vi "河内塔.vi"() -> ()   [LabVIEW 2016]
panel:
  in  "等待时间（毫秒）":u32=200
  out "二维图片":picture
  out "C":u8[](array[numeric])
  out "B":u8[](array[numeric])
  out "A":u8[](array[numeric])=[1, 2, 3]
  out "数组":cluster{"n":u8, "From":string, "To":string}[](array[cluster])=[{"n"=1, "From"="A", "To"="C"}, {"n"=2, "From"="A", "To"="B"}, {"n"=1, "From"="C", "To"="B"}, {"n"=3, "From"="A", "To"="C"}, {"n"=1, "From"="B", "To"="A"}, {"n"=2, "From"="B", "To"="C"}, {"n"=1, "From"="A", "To"="C"}]
  in  "N":u8=3 min=2 step=1
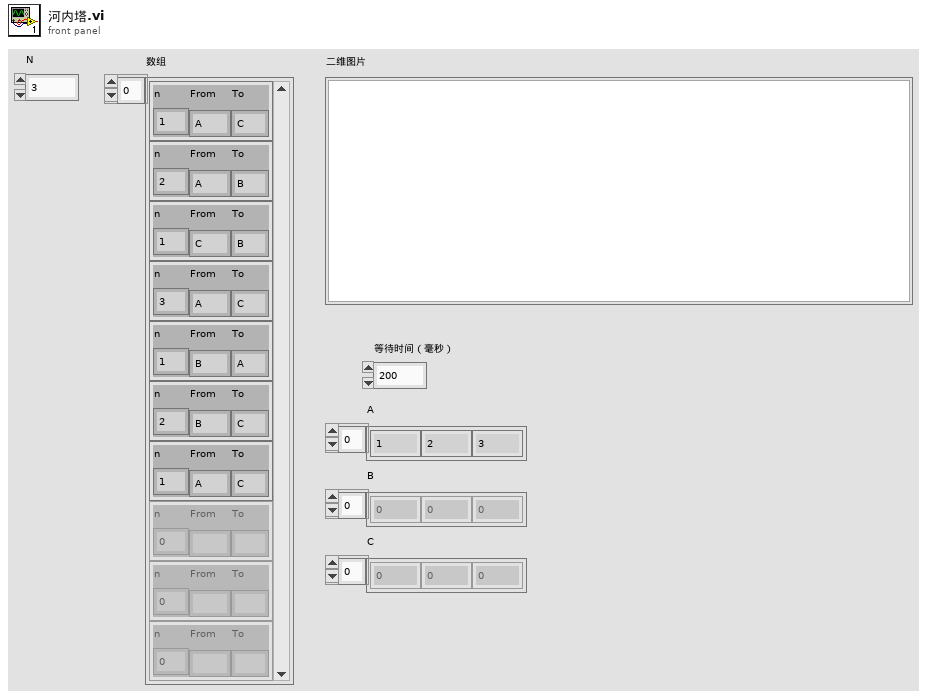
[diagram p1: front panel]
types:
  T1 = typedef "LVBoundsTypeDef.ctl" = cluster{"Width":u32, "Height":u32}
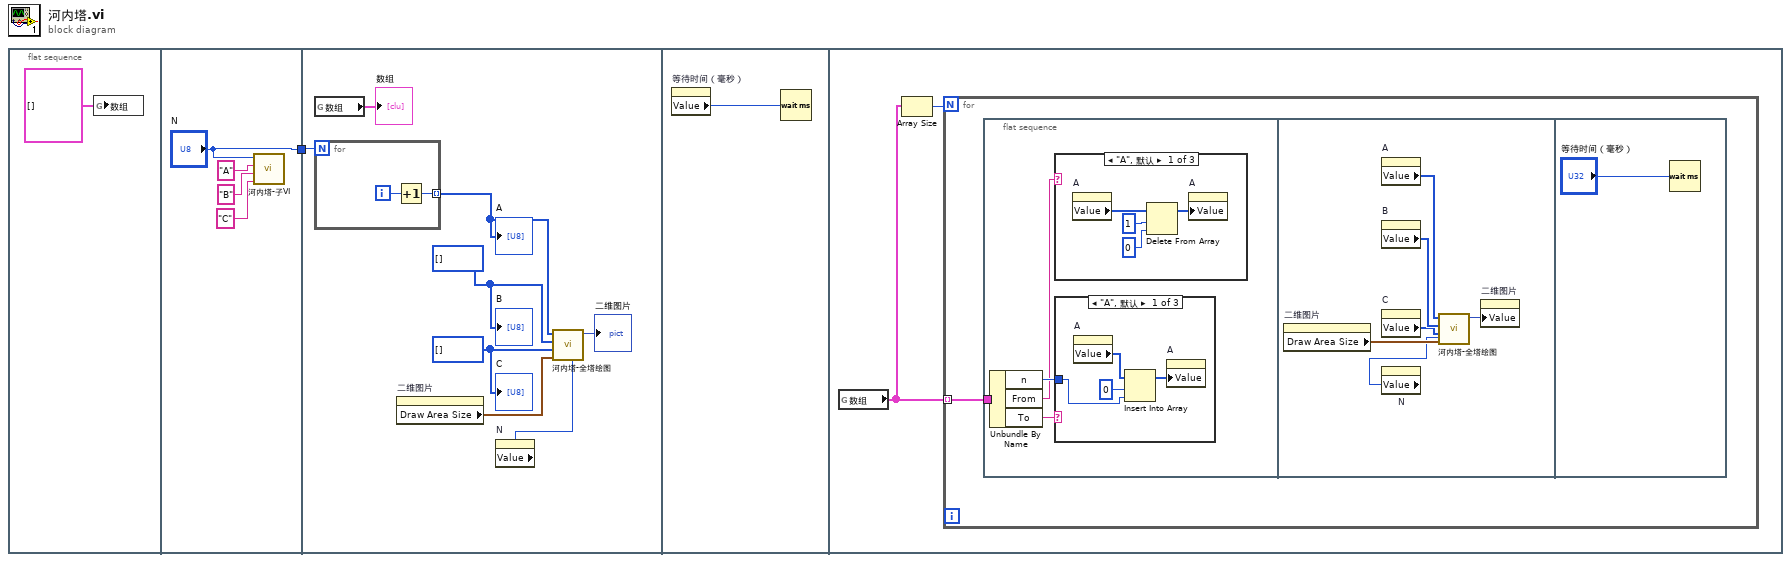
[diagram p0: block diagram]
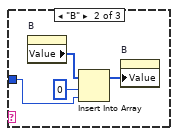
[diagram p2: hidden frame]
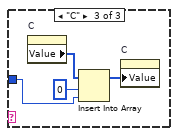
[diagram p3: hidden frame]
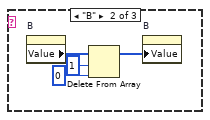
[diagram p4: hidden frame]
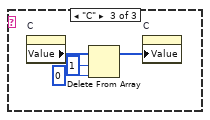
[diagram p5: hidden frame]
diagram:
  n1 = flat-sequence {
    tunnel: ["N"] -> w1
    tunnel: w1 -> [w14]
    frame #0 {
      n2 = global write "河内塔-全局.vi" "数组"(cluster{"n":u8, "From":string, "To":string}[] [] ("数组")) -> ()
    }
    frame #1 {
      n3 = call "河内塔-子VI.vi"("C"="C", "B"="B", "A"="A", "n"="N") -> ()  [unwired: 3 in]
    }
    frame #2 {
      w11 = u8[] [] ("C")
      w10 = u8[] [] ("C")
      n4 = global read "河内塔-全局.vi" "数组"() -> (→"数组":cluster{"n":u8, "From":string, "To":string}[])
      n5 = for {
        N: w14 -> [_]
        tunnel: [w16] -> w12 mode=indexing
        i -> [w15]
        n6 = Increment(x=w15) -> (x+1=w16:i32)
      }
      "A" <- w12
      n7 = property on="二维图片" class="Pict"() -> ("Draw Area Size"=w9:T1)  [unwired: 2 in, 2 out]
      n8 = property on="N" class="DigNum (严格)"() -> ("Value"=w7:u8)  [unwired: 2 in, 2 out]
      n9 = call "河内塔-全塔绘图.vi"("N"=w7, "绘图区域大小"=w9, "C"=w10, "B"=w11, "A"=w12) -> ("新图片"=→"二维图片":picture)  [unwired: 6 in]
      "C" <- w10
      "B" <- w11
    }
    frame #3 {
      n10 = property on="等待时间（毫秒）" class="DigNum (严格)"() -> ("Value"=w17:u32)  [unwired: 2 in, 2 out]
      n11 = Wait (ms)(milliseconds to wait=w17) -> ()  [unwired: 1 out]
    }
    frame #4 {
      n12 = global read "河内塔-全局.vi" "数组"() -> (w19:cluster{"n":u8, "From":string, "To":string}[])
      n13 = Array Size(array=w19) -> (size(s)=w18:i32)
      n14 = for {
        N: w18 -> [_]
        tunnel: w19 -> [w20] mode=indexing
        n15 = flat-sequence {
          tunnel: w20 -> [w21]
          frame #0 {
            n16 = Unbundle By Name(w21) -> ("n"=w24:u8, "From"=w22:string, "To"=w23:string)
            n17 = case shown="\"A\", 默认" w22 {
              frame "A", Default {
                n18 = property on="A" class="Arr (严格)"() -> ("Value"=w40:u8[])  [unwired: 2 in, 2 out]
                n19 = Delete From Array(array=w40, length=1 ("长度"), index=0 ("索引")) -> (array with subset deleted=w39:u8[])  [unwired: 1 out]
                n20 = property on="A" class="Arr (严格)"("Value"=w39) -> ()  [unwired: 2 in, 2 out]
              }
              frame "B" {
                n21 = property on="B" class="Arr (严格)"() -> ("Value"=w44:u8[])  [unwired: 2 in, 2 out]
                n22 = Delete From Array(array=w44, length=1 ("长度"), index=0 ("索引")) -> (array with subset deleted=w43:u8[])  [unwired: 1 out]
                n23 = property on="B" class="Arr (严格)"("Value"=w43) -> ()  [unwired: 2 in, 2 out]
              }
              frame "C" {
                n24 = property on="C" class="Arr (严格)"() -> ("Value"=w48:u8[])  [unwired: 2 in, 2 out]
                n25 = Delete From Array(array=w48, length=1 ("长度"), index=0 ("索引")) -> (array with subset deleted=w47:u8[])  [unwired: 1 out]
                n26 = property on="C" class="Arr (严格)"("Value"=w47) -> ()  [unwired: 2 in, 2 out]
              }
            }
            n27 = case shown="\"A\", 默认" w23 {
              tunnel: w24 -> [w25 w29 w36]
              frame "A", Default {
                n28 = property on="A" class="Arr (严格)"() -> ("Value"=w27:u8[])  [unwired: 2 in, 2 out]
                n29 = Insert Into Array(array=w27, index=0 ("索引"), new element=w25) -> (w28:u8[])
                n30 = property on="A" class="Arr (严格)"("Value"=w28) -> ()  [unwired: 2 in, 2 out]
              }
              frame "B" {
                n31 = property on="B" class="Arr (严格)"() -> ("Value"=w31:u8[])  [unwired: 2 in, 2 out]
                n32 = Insert Into Array(array=w31, index=0 ("索引"), new element=w29) -> (w32:u8[])
                n33 = property on="B" class="Arr (严格)"("Value"=w32) -> ()  [unwired: 2 in, 2 out]
              }
              frame "C" {
                n34 = property on="C" class="Arr (严格)"() -> ("Value"=w33:u8[])  [unwired: 2 in, 2 out]
                n35 = Insert Into Array(array=w33, index=0 ("索引"), new element=w36) -> (w34:u8[])
                n36 = property on="C" class="Arr (严格)"("Value"=w34) -> ()  [unwired: 2 in, 2 out]
              }
            }
          }
          frame #1 {
            n37 = property on="二维图片" class="Pict"() -> ("Draw Area Size"=w50:T1)  [unwired: 2 in, 2 out]
            n38 = property on="A" class="Arr (严格)"() -> ("Value"=w53:u8[])  [unwired: 2 in, 2 out]
            n39 = property on="B" class="Arr (严格)"() -> ("Value"=w52:u8[])  [unwired: 2 in, 2 out]
            n40 = property on="C" class="Arr (严格)"() -> ("Value"=w51:u8[])  [unwired: 2 in, 2 out]
            n41 = property on="N" class="DigNum (严格)"() -> ("Value"=w49:u8)  [unwired: 2 in, 2 out]
            n42 = call "河内塔-全塔绘图.vi"("N"=w49, "绘图区域大小"=w50, "C"=w51, "B"=w52, "A"=w53) -> ("新图片"=w54:picture)  [unwired: 6 in]
            n43 = property on="二维图片" class="Pict"("Value"=w54) -> ()  [unwired: 2 in, 2 out]
          }
          frame #2 {
            n44 = Wait (ms)(milliseconds to wait="等待时间（毫秒）") -> ()  [unwired: 1 out]
          }
        }
      }
    }
  }
